vi "CreateBackup.vi"(8 "error in":errorcluster, 10 "Backup path":path, 11 "Base Path":path) -> ()   [LabVIEW 2011]
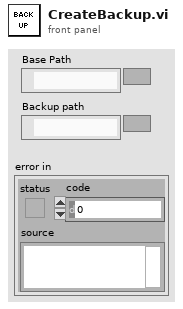
[diagram p1: front panel]
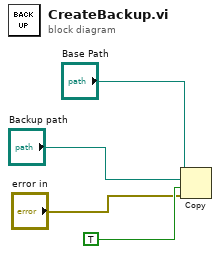
[diagram p0: block diagram]
diagram:
  n1 = Copy(8:"error in", 9:TRUE ("Treat LLBs as Folders?"), 10:"Backup path", 11:"Base Path") -> ()  [unwired: 1 in, 3 out]
